vi "RGBToU8Intensity.vi"(11 "Image Src":T1) -> (3 "Image Dst Out":T1)   [LabVIEW 2019]
uses:
  <vilib>/vision/Image Controls.llb/IMAQ Image.ctl
  <vilib>/vision/NI_Vision_Development_Module.lvlib
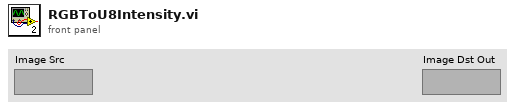
[diagram p1: front panel]
types:
  T1 = typedef "IMAQ Image.ctl" = refnum<image>
  T2 = typedef "Image Type" = u32
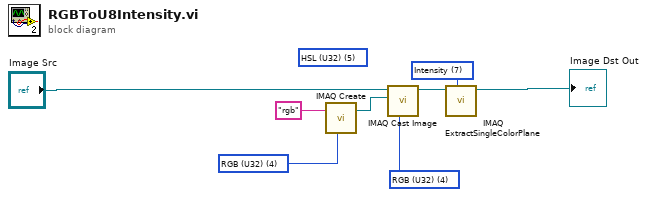
[diagram p0: block diagram]
diagram:
  w7 = 7 items=["Red", "Green", "Blue", "Hue", "Saturation", "Luminance", "Value", "Intensity"] ("Color Plane")
  w5 = T2 4 items=["Grayscale (U8)", "Grayscale (I16)", "Grayscale (SGL)", "Complex (CSG)", "RGB (U32)", "HSL (U32)", "RGB (U64)"] ("Image Type")
  w4 = T2 4 items=["Grayscale (U8)", "Grayscale (I16)", "Grayscale (SGL)", "Complex (CSG)", "RGB (U32)", "HSL (U32)", "RGB (U64)"] ("Image Type")
  (unwired) T2 5 items=["Grayscale (U8)", "Grayscale (I16)", "Grayscale (SGL)", "Complex (CSG)", "RGB (U32)", "HSL (U32)", "RGB (U64)"] ("Image Type")
  n1 = call "IMAQ Create"("Image Name"="rgb", "Image Type"=w4) -> ("New Image"=w2:T1)  [unwired: 2 in, 2 out]
  n2 = call "IMAQ Cast Image"("Image Type"=w5, "Image Dst"=w2, "Image Src"="Image Src") -> ("Image Dst Out"=w6:T1)  [unwired: 3 in, 5 out]
  n3 = call "IMAQ ExtractSingleColorPlane"("Color Plane"=w7, "Image Src"=w6) -> ("Image Dst Out"=→"Image Dst Out":T1)  [unwired: 2 in, 7 out]
